vi "Global 2.vi"() -> ()   [LabVIEW 2018]
panel:
  in  "Global index":dbl
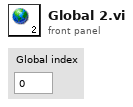
[diagram p1: front panel]
diagram:
